vi "Encode Byte.vi"(9 "Pixel Offset":i32, 10 "Byte To Encode":u8, 11 "Image In":u8[](array[numeric])) -> (3 "Image Out":u8[](array[numeric]))   [LabVIEW 2020]
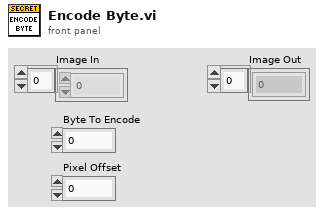
[diagram p1: front panel]
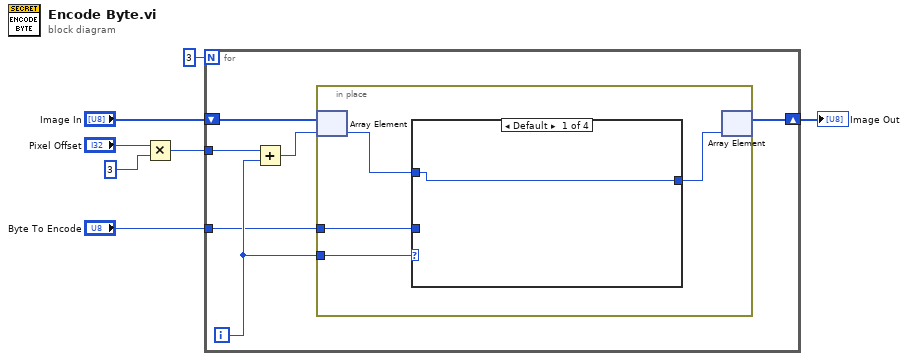
[diagram p0: block diagram]
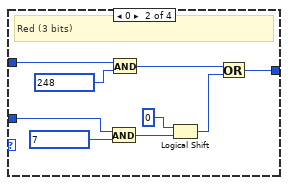
[diagram p2: hidden frame]
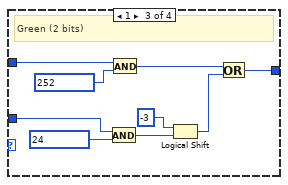
[diagram p3: hidden frame]
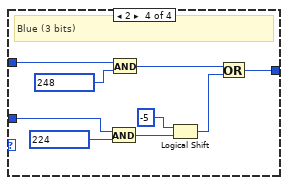
[diagram p4: hidden frame]
diagram:
  n1 = Multiply(x="Pixel Offset", y=3) -> (x*y=w1:i32)
  n2 = for {
    N: 3 -> [_]
    shift-right: [w12] -> w6
    shift-left: "Image In" -> [w13]
    tunnel: w1 -> [w11]
    tunnel: "Byte To Encode" -> [w8]
    i -> [w9]
    n3 = Add(x=w11, y=w9) -> (x+y=w10:i32)
    n4 = in-place {
      in-place-border: w9 -> [w15]
      in-place-border: w8 -> [w14]
      n5 = in-place-array #1(w13, w10) -> (w17:u8)
      n6 = case shown="Default" w15 {
        tunnel: w14 -> [_ w27 w36 w45]
        tunnel: w17 -> [w18 w25 w34 w43]
        tunnel: [w18 w19 w28 w37] -> w16
        frame Default {
        }
        frame 0 {
          # "Red (3 bits)"
          n7 = And(x=w27, y=u8 7) -> (x .and. y?=w22:u8)
          n8 = And(x=w25, y=u8 248) -> (x .and. y?=w23:u8)
          n9 = Logical Shift(y=i16 0, x=w22) -> (x << y=w21:u8)
          n10 = Or(x=w23, y=w21) -> (x .or. y?=w19:u8)
        }
        frame 1 {
          # "Green (2 bits)"
          n11 = And(x=w36, y=u8 24) -> (x .and. y?=w31:u8)
          n12 = And(x=w34, y=u8 252) -> (x .and. y?=w32:u8)
          n13 = Logical Shift(y=i16 -3, x=w31) -> (x << y=w30:u8)
          n14 = Or(x=w32, y=w30) -> (x .or. y?=w28:u8)
        }
        frame 2 {
          # "Blue (3 bits)"
          n15 = And(x=w45, y=u8 224) -> (x .and. y?=w40:u8)
          n16 = And(x=w43, y=u8 248) -> (x .and. y?=w41:u8)
          n17 = Logical Shift(y=i16 -5, x=w40) -> (x << y=w39:u8)
          n18 = Or(x=w41, y=w39) -> (x .or. y?=w37:u8)
        }
      }
      n19 = in-place-array #1(w16) -> (w12:u8[])  [unwired: 1 out]
    }
  }
  "Image Out" <- w6
